vi "Graph.vi"() -> ()   [LabVIEW 2011]
panel:
  out "output array":dbl[](array[numeric])
  out "appended array":dbl[][](array[numeric])
  out "DAQ Sample Plot":cluster{"xo":i32, "dx":i32, dbl[][]}(graph)
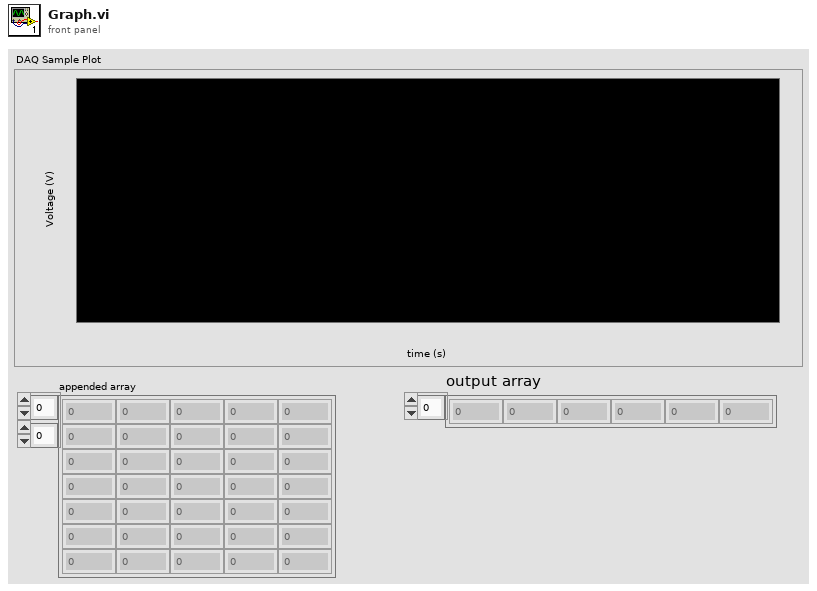
[diagram p1: front panel]
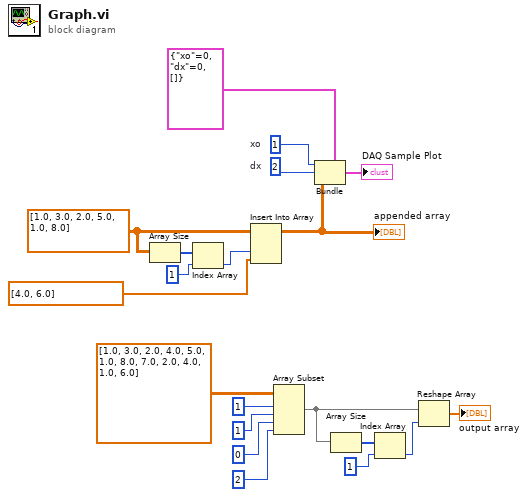
[diagram p0: block diagram]
diagram:
  w14 = dbl[][] [[1.0, 3.0, 2.0], [5.0, 1.0, 8.0]]
  w20 = 2  # dx
  w19 = 1  # xo
  n1 = Array Size(array=w14) -> (size(s)=w13:i32[])
  n2 = Index Array(array=w13, index=1) -> (element=w11:i32)
  n3 = Insert Into Array(array=w14, index (col)=w11, new element=dbl[] [4.0, 6.0]) -> (w15:dbl[][])  [unwired: 1 in]
  "appended array" <- w15
  n4 = Array Subset(array=dbl[][] [[1.0, 3.0, 2.0, 4.0], [5.0, 1.0, 8.0, 7.0], [2.0, 4.0, 1.0, 6.0]], index (row)=1 ("index"), length (row)=1 ("length"), index (col)=0 ("index"), length (col)=2 ("length")) -> (w5:dbl[][])
  n5 = Bundle(cluster=cluster{"xo":i32, "dx":i32, dbl[][]} {"xo"=0, "dx"=0, []}, "xo"=w19, "dx"=w20, w15) -> (→"DAQ Sample Plot":cluster{"xo":i32, "dx":i32, dbl[][]})
  n6 = Array Size(array=w5) -> (size(s)=w4:i32[])
  n7 = Index Array(array=w4, index=1) -> (element=w3:i32)
  n8 = Reshape Array(w5, w3) -> (→"output array":dbl[])
